vi "TurnOnOffSoleNoid.vi"(8 "error in (no error)":errorcluster, 10 "Boolean":bool, 11 "QUEUE IN":refnum<queue>) -> (0 "error out":errorcluster)   [LabVIEW 2017]
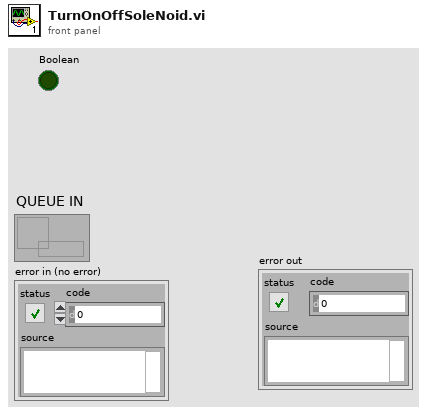
[diagram p1: front panel]
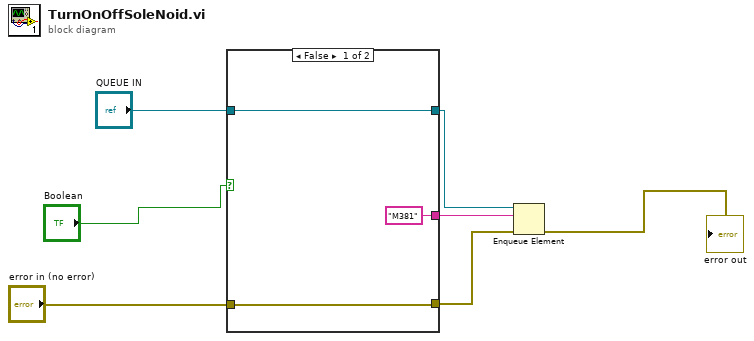
[diagram p0: block diagram]
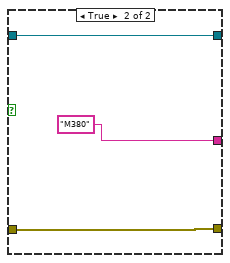
[diagram p2: hidden frame]
diagram:
  n1 = case shown="False" "Boolean" {
    tunnel: [w9 w13] -> w5
    tunnel: "QUEUE IN" -> [w9 w13]
    tunnel: [w8 w12] -> w3
    tunnel: "error in (no error)" -> [w8 w12]
    tunnel: ["M381" ("element") "M380" ("element")] -> w1
    frame False {
    }
    frame True {
    }
  }
  n2 = Enqueue Element(queue=w5, element=w1, error in (no error)=w3) -> (error out=→"error out":errorcluster)  [unwired: 1 in, 2 out]
